vi "ILAB_IsLoaded.vi"(3 "name":string) -> (0 "status":bool)   [LabVIEW 2009]
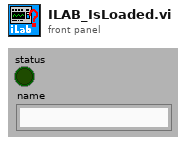
[diagram p1: front panel]
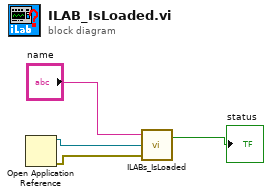
[diagram p0: block diagram]
diagram:
  n1 = Open Application Reference() -> (0:w4:errorcluster, 3:w3:refnum<vi>)  [unwired: 1 in, 3 out]
  n2 = call "ILABs_IsLoaded.vi"("error in (no error)"=w4, "appRef"=w3, "name"="name") -> ("status"=→"status":bool)  [unwired: 1 out]
